vi "IMU Parsing (Euler angle, Acceleration).vi"(2 "IMU Data":string) -> (5 "IMU_Roll":dbl, 6 "IMU_Pitch":dbl, 7 "IMU_Yaw":dbl, 8 "IMU Raw ax":dbl)   [LabVIEW 2016]
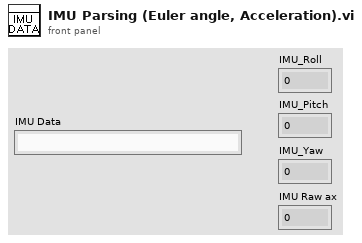
[diagram p1: front panel]
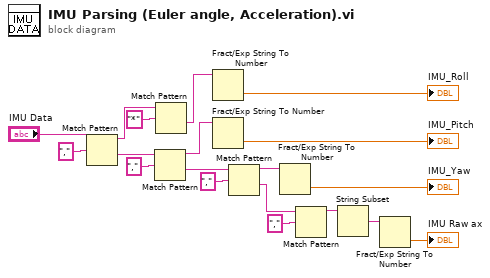
[diagram p0: block diagram]
diagram:
  n1 = Match Pattern(string="IMU Data", regular expression="," ("정규식")) -> (before substring=w14:string, after substring=w12:string)  [unwired: 1 in, 2 out]
  n2 = Match Pattern(string=w12, regular expression="," ("정규식")) -> (before substring=w17:string, after substring=w13:string)  [unwired: 1 in, 2 out]
  n3 = Match Pattern(string=w14, regular expression="*" ("정규식")) -> (after substring=w16:string)  [unwired: 1 in, 3 out]
  n4 = Fract/Exp String To Number(string=w16) -> (number=→"IMU_Roll":dbl)  [unwired: 3 in, 1 out]
  n5 = Fract/Exp String To Number(string=w17) -> (number=→"IMU_Pitch":dbl)  [unwired: 3 in, 1 out]
  n6 = Match Pattern(string=w13, regular expression="," ("정규식")) -> (before substring=w18:string, after substring=w7:string)  [unwired: 1 in, 2 out]
  n7 = Fract/Exp String To Number(string=w18) -> (number=→"IMU_Yaw":dbl)  [unwired: 3 in, 1 out]
  n8 = Match Pattern(string=w7, regular expression="," ("정규식")) -> (before substring=w6:string)  [unwired: 1 in, 3 out]
  n9 = String Subset(string=w6) -> (substring=w5:string)  [unwired: 2 in]
  n10 = Fract/Exp String To Number(string=w5) -> (number=→"IMU Raw ax":dbl)  [unwired: 3 in, 1 out]
